vi "Teleop.vi"(10 "Match Info":T1={"Autonomous Elapsed Seconds"=0.0, "TeleOp Elapsed Seconds"=0.0, "Disabled Elapsed Seconds"=0.0, "Visited Autonomous"=FALSE, "Visited TeleOp"=FALSE, "Visited Disabled"=FALSE, "Autonomous Settings"={"Autonomous Style"=enum."Independent", "VI Refnum"=refnum}}, 11 "Call Context":T2) -> ()   [LabVIEW 2017]
doc: "This VI is called for each TeleOp packet received from the DS where the robot is not disabled. It is often used to read from the joysticks and update I/O or to update setpoints for timed control loops. It should complete and return within 20 milliseconds or it may miss DS packets."
uses:
  <vilib>/Rock Robotics/WPI/DriverStation/WPI_DriverStationDerivedRobotMode.ctl
  <vilib>/Rock Robotics/WPI/DriverStation/WPI_DriverStationMatch Info.ctl
  <vilib>/Rock Robotics/WPI/Solenoid/WPI_SolenoidValue.ctl
  <vilib>/Rock Robotics/WPI/Utilities/WPI_GetSetVariantRefNum.vi
  Desktop/2018 FINAL/E/2018 FINAL/C/Users/admin/Documents/LabVIEW Data/2018 FINAL CODE/Robot Global Data.vi
  <vilib>/Rock Robotics/WPI/Solenoid/WPI_SolenoidSetEnum.vi
  <vilib>/addons/control/pid/pid.llb/PID (DBL).vi
  <vilib>/addons/control/pid/NI_PID_pid.lvlib
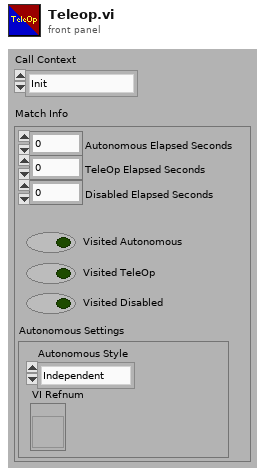
[diagram p1: front panel]
types:
  T1 = typedef "WPI_DriverStationMatch Info.ctl" = cluster{"Autonomous Elapsed Seconds":dbl, "TeleOp Elapsed Seconds":dbl, "Disabled Elapsed Seconds":dbl, "Visited Autonomous":bool, "Visited TeleOp":bool, "Visited Disabled":bool, "Autonomous Settings":cluster{"Autonomous Style":enum16{"Iterative", "Independent"}, "VI Refnum":refnum<vi>}}
  T2 = typedef "WPI_DriverStationDerivedRobotMode.ctl" = enum16{"Init", "Execute", "Stop"}
  T3 = cluster{"proportional gain (Kc)":dbl, "integral time (Ti, min)":dbl, "derivative time (Td, min)":dbl}
  T4 = enum16{"NONE", "LEVEL 1", "LEVEL 2", "LEVEL 3", "LEVEL 4"}
  T5 = typedef "WPI_SolenoidValue.ctl" = enum16{"Off", "On", "Forward", "Reverse"}
  T6 = typedef "WPI_JoystickDevRef.ctl" = cluster{"Device":T7}
  T7 = typedef "WPI_JoystickDeviceEnum.ctl" = enum16{"USB 0", "USB 1", "USB 2", "USB 3", "USB 4", "USB 5"}
  T8 = typedef "WPI_RobotDriveDevRef.ctl" = cluster{"DevStatus":errorcluster, "Motors[]":T9[], "Square Inputs":bool, "Max Output":dbl}
  T9 = typedef "WPI_MotorControlDeviceRef.ctl" = cluster{"DeviceStatus":errorcluster, "Type":T10, "PWM":cluster{"PWM Channel":T11, "DeadBand":T12}, "CAN":cluster{"Device Number":u8, "SetOutput VI Ref":variant, "GetOutput VI Ref":variant, "Enable VI Ref":variant, "Disable VI Ref":variant, "Data":variant}, "Invert":bool, "DIO PWM":cluster{"PWM \"Enable\" Channel":T11, "DIOChannel":T13, "PWM Rate":dbl}}
  T10 = typedef "WPI_MotorControlType.ctl" = enum16{"PWM", "CAN", "DIO PWM"}
  T11 = typedef "FPGA_DIOPWMChannel.ctl" = enum8{"PWM 0", "PWM 1", "PWM 2", "PWM 3", "PWM 4", "PWM 5", "PWM 6", "PWM 7", "PWM 8", "PWM 9", "PWM MXP 0", "PWM MXP 1", "PWM MXP 2", "PWM MXP 3", "PWM MXP 4", "PWM MXP 5", "PWM MXP 6", "PWM MXP 7", "PWM MXP 8", "PWM MXP 9", "Invalid"}
  T12 = typedef "WPI_PWMDeadband.ctl" = cluster{"Name":string, "maxPositivePwm":i32, "minPositivePwm":i32, "centerPwm":i32, "maxNegativePwm":i32, "minNegativePwm":i32, "angularRange":u16}
  T13 = typedef "FPGA_DIOChannel.ctl" = enum8{"DIO 0", "DIO 1", "DIO 2", "DIO 3", "DIO 4", "DIO 5", "DIO 6", "DIO 7", "DIO 8", "DIO 9", "DIO MXP 0", "DIO MXP 1", "DIO MXP 2", "DIO MXP 3", "DIO MXP 4", "DIO MXP 5", "DIO MXP 6", "DIO MXP 7", "DIO MXP 8", "DIO MXP 9", "DIO MXP 10", "DIO MXP 11", "DIO MXP 12", "DIO MXP 13", "DIO MXP 14", "DIO MXP 15", "SPI Port CS1", "SPI Port CS2", "SPI Port CS3", "SPI Port MISO", "SPI Port MOSI", "Invalid"}
  T14 = typedef "WPI_PotentiometerDevRef.ctl" = cluster{"DevStatus":errorcluster, "Analog Channel":T15, "Invert Output":bool}
  T15 = typedef "FPGA_AIChannel.ctl" = enum8{"AI 0", "AI 1", "AI 2", "AI 3", "AI MXP 0", "AI MXP 1", "AI MXP 2", "AI MXP 3", "Invalid"}
  T16 = typedef "WPI_SolenoidDevRef.ctl" = cluster{"DevStatus":errorcluster, "Pneumatics Control Module":u8, "Forward Solenoid Channel":T17, "Reverse Solenoid Channel":T17}
  T17 = typedef "WPI_SolenoidChannel.ctl" = enum8{"Solenoid 0", "Solenoid 1", "Solenoid 2", "Solenoid 3", "Solenoid 4", "Solenoid 5", "Solenoid 6", "Solenoid 7", "Invalid"}
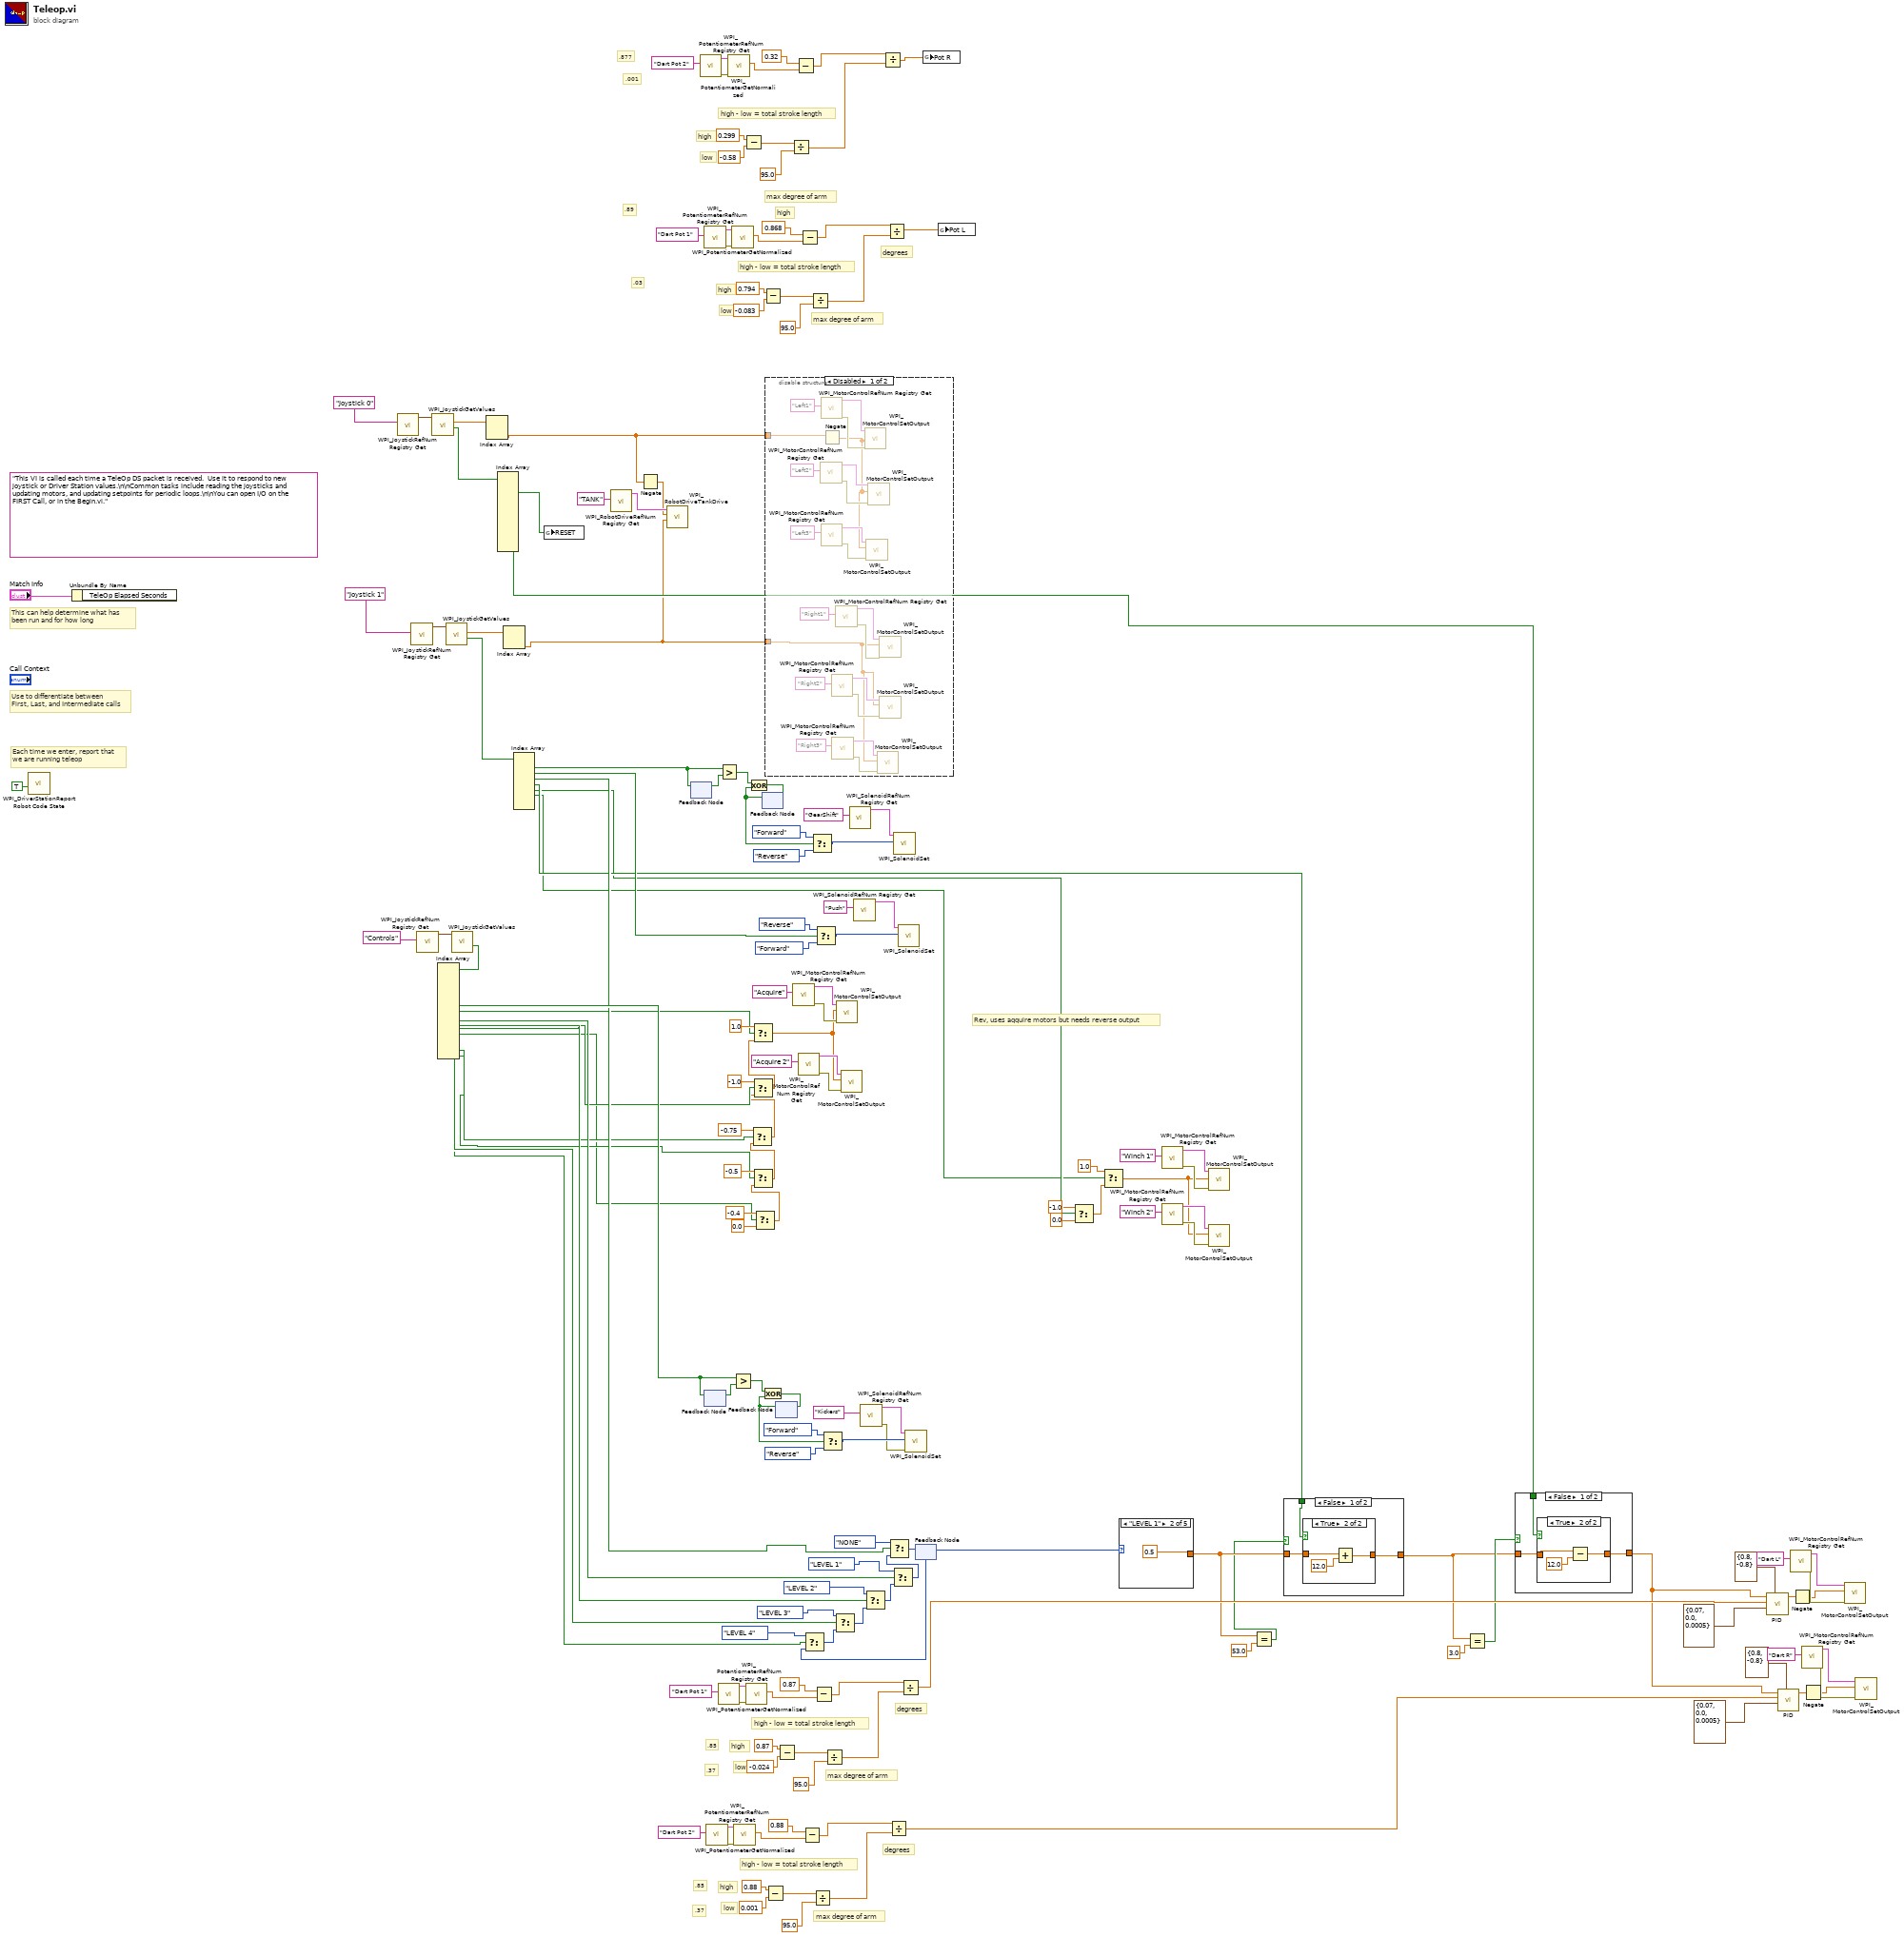
[diagram p0: block diagram]
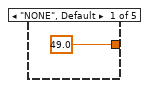
[diagram p7: hidden frame]
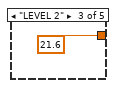
[diagram p8: hidden frame]
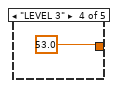
[diagram p9: hidden frame]
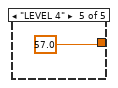
[diagram p10: hidden frame]
diagram:
  (unwired) "This VI is called each time a TeleOp DS packet is received.  Use it to respond to new joystick or Driver Station values.\n\nCommon tasks include reading the joysticks and updating motors, and updating setpoints for periodic loops.\n\nYou can open I/O on the FIRST Call, or in the Begin.vi."
  # ".03"
  # ".89"
  # ".001"
  # ".877"
  # ".37"
  # ".85"
  # "max degree of arm"
  # "degrees"
  # "low"
  # "high"
  # "high - low = total stroke length"
  # ".37"
  # ".85"
  # "max degree of arm"
  # "degrees"
  # "low"
  # "high"
  # "high - low = total stroke length"
  # "max degree of arm"
  # "max degree of arm"
  # "low"
  # "high"
  # "high - low = total stroke length"
  # "degrees"
  # "low"
  # "high"
  # "high - low = total stroke length"
  # "high"
  # "Rev, uses aqquire motors but needs reverse output"
  # "Each time we enter, report that\nwe are running teleop"
  # "Use to differentiate between\nFirst, Last, and Intermediate calls"
  # "This can help determine what has\nbeen run and for how long"
  n1 = call <vilib>:"WPI_DriverStationReport Robot Code State.vi"("TeleOp"=TRUE ("Autonomous")) -> ()  [unwired: 10 in, 1 out]
  n2 = Unbundle By Name("Match Info") -> ()  [unwired: 1 out]
  n3 = call <vilib>:"WPI_JoystickRefNum Registry Get.vi"("refnum name"="Joystick 0") -> ("JoystickDevRef"=w165:T6)  [unwired: 1 in, 9 out]
  n4 = call <vilib>:"WPI_JoystickRefNum Registry Get.vi"("refnum name"="Joystick 1") -> ("JoystickDevRef"=w162:T6)  [unwired: 1 in, 9 out]
  n5 = call <vilib>:"WPI_JoystickRefNum Registry Get.vi"("refnum name"="Controls") -> ("JoystickDevRef"=w143:T6)  [unwired: 1 in, 9 out]
  n6 = call <vilib>:"WPI_JoystickGetValues.vi"("JoystickDevRef"=w165) -> ("Buttons"=w61:bool[], "Axes"=w164:dbl[])  [unwired: 6 in, 3 out]
  n7 = call <vilib>:"WPI_JoystickGetValues.vi"("JoystickDevRef"=w162) -> ("Buttons"=w160:bool[], "Axes"=w161:dbl[])  [unwired: 6 in, 3 out]
  n8 = call <vilib>:"WPI_JoystickGetValues.vi"("JoystickDevRef"=w143) -> ("Buttons"=w142:bool[])  [unwired: 6 in, 4 out]
  n9 = Index Array(array=w142) -> (element #3=w34:bool, element #4=w89:bool, element #5=w88:bool, element #6=w86:bool, element #7=w24:bool, element #10=w17:bool, element #11=w7:bool, element #12=w93:bool, element #14=w12:bool, element #15=w11:bool)  [unwired: 15 in, 5 out]
  n10 = Index Array(array=w164) -> (element #2=w3:dbl)  [unwired: 2 in, 1 out]
  n11 = Index Array(array=w61) -> (element #2=w55:bool, element #4=w60:bool)  [unwired: 12 in, 10 out]
  n12 = Index Array(array=w161) -> (element #2=w4:dbl)  [unwired: 2 in, 1 out]
  n13 = Index Array(array=w160) -> (element #1=w155:bool, element #2=w69:bool, element #3=w70:bool, element #4=w68:bool, element #5=w58:bool, element #6=w29:bool)  [unwired: 8 in, 2 out]
  n14 = global write "Robot Global Data.vi" "RESET"(w55) -> ()
  n15 = call <vilib>:"WPI_RobotDriveRefNum Registry Get.vi"("refnum name"="TANK") -> ("RobotDriveDevRef"=w6:T8)  [unwired: 9 in, 1 out]
  n16 = Negate(x=w3) -> (-x=w2:dbl)
  n17 = call <vilib>:"WPI_RobotDriveTankDrive.vi"("Right axis value"=w4, "Left axis value"=w2, "RobotDriveDevRef"=w6) -> ()  [unwired: 6 in, 3 out]
  n18 = feedback #1() -> (w156:bool)  [unwired: 1 in]
  n19 = feedback-in #1(w155) -> ()
  n20 = call <vilib>:"WPI_PotentiometerRefNum Registry Get.vi"("refnum name"="Dart Pot 2") -> ("error out"=w123:errorcluster, "PotDevRef"=w122:T14)  [unwired: 9 in]
  n21 = call <vilib>:"WPI_PotentiometerRefNum Registry Get.vi"("refnum name"="Dart Pot 1") -> ("error out"=w128:errorcluster, "PotDevRef"=w127:T14)  [unwired: 9 in]
  n22 = feedback #2() -> (w87:bool)  [unwired: 1 in]
  n23 = feedback-in #2(w86) -> ()
  n24 = call <vilib>:"WPI_PotentiometerRefNum Registry Get.vi"("refnum name"="Dart Pot 2") -> ("error out"=w46:errorcluster, "PotDevRef"=w45:T14)  [unwired: 9 in]
  n25 = call <vilib>:"WPI_PotentiometerRefNum Registry Get.vi"("refnum name"="Dart Pot 1") -> ("error out"=w105:errorcluster, "PotDevRef"=w104:T14)  [unwired: 9 in]
  n26 = Greater?(x=w155, y=w156) -> (0:w159:bool)
  n27 = call <vilib>:"WPI_PotentiometerGetNormalized.vi"("error in"=w123, "PotDevRef"=w122) -> ("Normalized Value"=w1:dbl)  [unwired: 7 in, 2 out]
  n28 = call <vilib>:"WPI_PotentiometerGetNormalized.vi"("error in"=w128, "PotDevRef"=w127) -> ("Normalized Value"=w118:dbl)  [unwired: 7 in, 2 out]
  n29 = Greater?(x=w86, y=w87) -> (0:w132:bool)
  n30 = call <vilib>:"WPI_PotentiometerGetNormalized.vi"("error in"=w46, "PotDevRef"=w45) -> ("Normalized Value"=w41:dbl)  [unwired: 7 in, 2 out]
  n31 = Subtract(x=0.299 ("y"), y=-0.58) -> (x-y=w110:dbl)
  n32 = call <vilib>:"WPI_PotentiometerGetNormalized.vi"("error in"=w105, "PotDevRef"=w104) -> ("Normalized Value"=w100:dbl)  [unwired: 7 in, 2 out]
  n33 = Select(t=-0.4, s=w7, f=0.0) -> (s? t:f=w8:dbl)
  n34 = Select(t=-0.5, s=w11, f=w8) -> (s? t:f=w13:dbl)
  n35 = Select(t=-0.75, s=w12, f=w13) -> (s? t:f=w14:dbl)
  n36 = Select(t=-1.0, s=w17, f=w14) -> (s? t:f=w20:dbl)
  n37 = Select(t=1.0, s=w24, f=w20) -> (s? t:f=w18:dbl)
  n38 = feedback #3() -> (w157:bool)  [unwired: 1 in]
  n39 = Exclusive Or(1:w157, 2:w159) -> (0:w158:bool)
  n40 = feedback-in #3(w158) -> ()
  n41 = Subtract(x=0.794 ("y"), y=-0.083) -> (x-y=w115:dbl)
  n42 = Subtract(x=0.88 ("y"), y=0.001) -> (x-y=w38:dbl)
  n43 = disable-structure shown="Disabled" {
    disable-tunnel: w3 -> [w183 _]
    disable-tunnel: w4 -> [w176 _]
    frame Disabled {
      n44 = call <vilib>:"WPI_MotorControlRefNum Registry Get.vi"("refnum name"="Left2") -> ("error out"=w173:errorcluster, "MotorControlDevRef"=w174:T9)  [unwired: 9 in]
      n45 = call <vilib>:"WPI_MotorControlRefNum Registry Get.vi"("refnum name"="Left1") -> ("error out"=w184:errorcluster, "MotorControlDevRef"=w188:T9)  [unwired: 9 in]
      n46 = call <vilib>:"WPI_MotorControlRefNum Registry Get.vi"("refnum name"="Left3") -> ("error out"=w170:errorcluster, "MotorControlDevRef"=w171:T9)  [unwired: 9 in]
      n47 = Negate(x=w183) -> (-x=w169:dbl)
      n48 = call <vilib>:"WPI_MotorControlRefNum Registry Get.vi"("refnum name"="Right2") -> ("error out"=w180:errorcluster, "MotorControlDevRef"=w181:T9)  [unwired: 9 in]
      n49 = call <vilib>:"WPI_MotorControlRefNum Registry Get.vi"("refnum name"="Right3") -> ("error out"=w177:errorcluster, "MotorControlDevRef"=w178:T9)  [unwired: 9 in]
      n50 = call <vilib>:"WPI_MotorControlRefNum Registry Get.vi"("refnum name"="Right1") -> ("error out"=w185:errorcluster, "MotorControlDevRef"=w186:T9)  [unwired: 9 in]
      n51 = call <vilib>:"WPI_MotorControlSetOutput.vi"("error in (no error)"=w184, "Output"=w169, "MotorControlDevRef"=w188) -> ()  [unwired: 6 in, 3 out]
      n52 = call <vilib>:"WPI_MotorControlSetOutput.vi"("error in (no error)"=w170, "Output"=w169, "MotorControlDevRef"=w171) -> ()  [unwired: 6 in, 3 out]
      n53 = call <vilib>:"WPI_MotorControlSetOutput.vi"("error in (no error)"=w173, "Output"=w169, "MotorControlDevRef"=w174) -> ()  [unwired: 6 in, 3 out]
      n54 = call <vilib>:"WPI_MotorControlSetOutput.vi"("error in (no error)"=w177, "Output"=w176, "MotorControlDevRef"=w178) -> ()  [unwired: 6 in, 3 out]
      n55 = call <vilib>:"WPI_MotorControlSetOutput.vi"("error in (no error)"=w185, "Output"=w176, "MotorControlDevRef"=w186) -> ()  [unwired: 6 in, 3 out]
      n56 = call <vilib>:"WPI_MotorControlSetOutput.vi"("error in (no error)"=w180, "Output"=w176, "MotorControlDevRef"=w181) -> ()  [unwired: 6 in, 3 out]
    }
    frame Enabled {
    }
  }
  n57 = feedback #4() -> (w130:bool)  [unwired: 1 in]
  n58 = Exclusive Or(1:w130, 2:w132) -> (0:w131:bool)
  n59 = feedback-in #4(w131) -> ()
  n60 = Subtract(x=0.87 ("y"), y=-0.024) -> (x-y=w97:dbl)
  n61 = Divide(x=w110, y=95.0) -> (x/y=w108:dbl)
  n62 = call <vilib>:"WPI_MotorControlRefNum Registry Get.vi"("refnum name"="Acquire") -> ("error out"=w26:errorcluster, "MotorControlDevRef"=w27:T9)  [unwired: 9 in]
  n63 = Subtract(x=0.32 ("y"), y=w1) -> (x-y=w119:dbl)
  n64 = call <vilib>:"WPI_MotorControlRefNum Registry Get.vi"("refnum name"="Acquire 2") -> ("error out"=w21:errorcluster, "MotorControlDevRef"=w22:T9)  [unwired: 9 in]
  n65 = Subtract(x=0.868 ("y"), y=w118) -> (x-y=w124:dbl)
  n66 = Subtract(x=0.88 ("y"), y=w41) -> (x-y=w42:dbl)
  n67 = Divide(x=w115, y=95.0) -> (x/y=w113:dbl)
  n68 = Select(t=WPI_SolenoidValue."Forward" ("Value"), s=w157, f=WPI_SolenoidValue."Reverse" ("Value")) -> (s? t:f=w150:T5)
  n69 = Divide(x=w38, y=95.0) -> (x/y=w36:dbl)
  n70 = Subtract(x=0.87 ("y"), y=w100) -> (x-y=w101:dbl)
  n71 = Select(t=WPI_SolenoidValue."Reverse" ("Value"), s=w69, f=WPI_SolenoidValue."Forward" ("Value")) -> (s? t:f=w145:T5)
  n72 = Select(t=WPI_SolenoidValue."Forward" ("Value"), s=w130, f=WPI_SolenoidValue."Reverse" ("Value")) -> (s? t:f=w135:T5)
  n73 = Divide(x=w97, y=95.0) -> (x/y=w95:dbl)
  n74 = call <vilib>:"WPI_MotorControlSetOutput.vi"("error in (no error)"=w26, "Output"=w18, "MotorControlDevRef"=w27) -> ()  [unwired: 6 in, 3 out]
  n75 = call <vilib>:"WPI_MotorControlSetOutput.vi"("error in (no error)"=w21, "Output"=w18, "MotorControlDevRef"=w22) -> ()  [unwired: 6 in, 3 out]
  n76 = call <vilib>:"WPI_SolenoidRefNum Registry Get.vi"("refnum name"="GearShift") -> ("SolenoidDevRef"=w153:T16)  [unwired: 9 in, 1 out]
  n77 = call <vilib>:"WPI_SolenoidRefNum Registry Get.vi"("refnum name"="Push") -> ("SolenoidDevRef"=w148:T16)  [unwired: 9 in, 1 out]
  n78 = call <vilib>:"WPI_SolenoidRefNum Registry Get.vi"("refnum name"="Kickers") -> ("error out"=w133:errorcluster, "SolenoidDevRef"=w134:T16)  [unwired: 9 in]
  n79 = Divide(x=w119, y=w108) -> (x/y=w106:dbl)
  n80 = Divide(x=w124, y=w113) -> (x/y=w107:dbl)
  n81 = Divide(x=w42, y=w36) -> (x/y=w35:dbl)
  n82 = call-poly <vilib>:"WPI_SolenoidSet.vi"("Value"=w150, "SolenoidDevRef"=w153) -> ()  [unwired: 8 in, 2 out]
  n83 = call-poly <vilib>:"WPI_SolenoidSet.vi"("Value"=w145, "SolenoidDevRef"=w148) -> ()  [unwired: 8 in, 2 out]
  n84 = Divide(x=w101, y=w95) -> (x/y=w94:dbl)
  n85 = call-poly <vilib>:"WPI_SolenoidSet.vi"("error in (no error)"=w133, "Value"=w135, "SolenoidDevRef"=w134) -> ()  [unwired: 7 in, 2 out]
  n86 = feedback #5() -> (w71:T4)  [unwired: 1 in]
  n87 = Select(t=T4."LEVEL 4", s=w88, f=w71) -> (s? t:f=w90:T4)
  n88 = Select(t=T4."LEVEL 3", s=w89, f=w90) -> (s? t:f=w91:T4)
  n89 = Select(t=T4."LEVEL 2", s=w34, f=w91) -> (s? t:f=w92:T4)
  n90 = Select(t=T4."LEVEL 1", s=w93, f=w92) -> (s? t:f=w76:T4)
  n91 = Select(t=T4."NONE", s=w70, f=w76) -> (s? t:f=w78:T4)
  n92 = feedback-in #5(w78) -> ()
  n93 = global write "Robot Global Data.vi" "Pot R"(w106) -> ()
  n94 = global write "Robot Global Data.vi" "Pot L"(w107) -> ()
  n95 = Select(t=-1.0, s=w58, f=0.0) -> (s? t:f=w59:dbl)
  n96 = Select(t=1.0, s=w29, f=w59) -> (s? t:f=w30:dbl)
  n97 = case shown="\"LEVEL 1\"" w71 {
    tunnel: [49.0 0.5 21.6 53.0 57.0] -> w67
    frame "NONE", Default {
    }
    frame "LEVEL 1" {
    }
    frame "LEVEL 2" {
    }
    frame "LEVEL 3" {
    }
    frame "LEVEL 4" {
    }
  }
  n98 = call <vilib>:"WPI_MotorControlRefNum Registry Get.vi"("refnum name"="Winch 1") -> ("error out"=w138:errorcluster, "MotorControlDevRef"=w139:T9)  [unwired: 9 in]
  n99 = call <vilib>:"WPI_MotorControlRefNum Registry Get.vi"("refnum name"="Winch 2") -> ("error out"=w31:errorcluster, "MotorControlDevRef"=w32:T9)  [unwired: 9 in]
  n100 = call <vilib>:"WPI_MotorControlSetOutput.vi"("error in (no error)"=w138, "Output"=w30, "MotorControlDevRef"=w139) -> ()  [unwired: 6 in, 3 out]
  n101 = call <vilib>:"WPI_MotorControlSetOutput.vi"("error in (no error)"=w31, "Output"=w30, "MotorControlDevRef"=w32) -> ()  [unwired: 6 in, 3 out]
  n102 = Equal?(x=w67, y=53.0) -> (x = y?=w65:bool)
  n103 = case shown="False" w65 {
    tunnel: w68 -> [w195 _]
    tunnel: [w196 w202] -> w62
    tunnel: w67 -> [w197 w202]
    frame False {
      n104 = case shown="True" w195 {
        tunnel: [w198 w200] -> w196
        tunnel: w197 -> [w198 w199]
        frame False {
        }
        frame True {
          n105 = Add(x=w199, y=12.0) -> (x+y=w200:dbl)
        }
      }
    }
    frame True {
    }
  }
  n106 = Equal?(x=w62, y=3.0) -> (x = y?=w63:bool)
  n107 = case shown="False" w63 {
    tunnel: w62 -> [w205 w210]
    tunnel: [w204 w210] -> w47
    tunnel: w60 -> [w203 _]
    frame False {
      n108 = case shown="True" w203 {
        tunnel: w205 -> [w206 w209]
        tunnel: [w206 w207] -> w204
        frame False {
        }
        frame True {
          n109 = Subtract(x=w209, y=12.0) -> (x-y=w207:dbl)
        }
      }
    }
    frame True {
    }
  }
  n110 = call-poly <vilib>:"PID.vi"("output range"=cluster{"output high":dbl, "output low":dbl} {"output high"=0.8, "output low"=-0.8}, "PID gains"=T3 {"proportional gain (Kc)"=0.07, "integral time (Ti, min)"=0.0, "derivative time (Td, min)"=0.0005}, "process variable"=w94, "setpoint"=w47) -> ("output"=w83:dbl)  [unwired: 6 in, 1 out]
  n111 = call-poly <vilib>:"PID.vi"("output range"=cluster{"output high":dbl, "output low":dbl} {"output high"=0.8, "output low"=-0.8}, "PID gains"=T3 {"proportional gain (Kc)"=0.07, "integral time (Ti, min)"=0.0, "derivative time (Td, min)"=0.0005}, "process variable"=w35, "setpoint"=w47) -> ("output"=w52:dbl)  [unwired: 6 in, 1 out]
  n112 = call <vilib>:"WPI_MotorControlRefNum Registry Get.vi"("refnum name"="Dart L") -> ("error out"=w84:errorcluster, "MotorControlDevRef"=w81:T9)  [unwired: 9 in]
  n113 = Negate(x=w83) -> (-x=w82:dbl)
  n114 = call <vilib>:"WPI_MotorControlRefNum Registry Get.vi"("refnum name"="Dart R") -> ("error out"=w53:errorcluster, "MotorControlDevRef"=w50:T9)  [unwired: 9 in]
  n115 = Negate(x=w52) -> (-x=w51:dbl)
  n116 = call <vilib>:"WPI_MotorControlSetOutput.vi"("error in (no error)"=w84, "Output"=w82, "MotorControlDevRef"=w81) -> ()  [unwired: 6 in, 3 out]
  n117 = call <vilib>:"WPI_MotorControlSetOutput.vi"("error in (no error)"=w53, "Output"=w51, "MotorControlDevRef"=w50) -> ()  [unwired: 6 in, 3 out]
